vi "LVFunction_Determine if config file needs installer.vi"(0 "Config file path":path, 5 "Product version":string, 7 "Product name":string, 11 "error in (no error)":errorcluster) -> (4 "Config file path (dup)":path, 6 "must install":bool, 15 "error out":errorcluster)   [LabVIEW 2020]
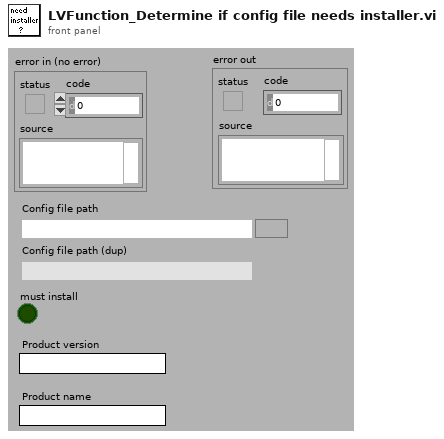
[diagram p1: front panel]
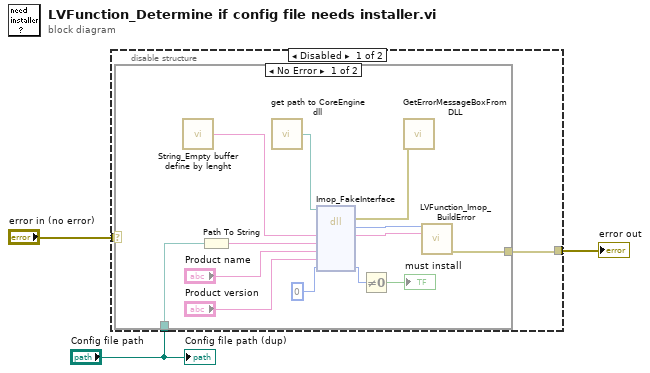
[diagram p0: block diagram]
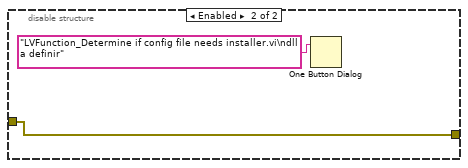
[diagram p3: hidden frame]
diagram:
  n1 = disable-structure shown="Disabled" {
    disable-tunnel: "error in (no error)" -> [w6 w22]
    disable-tunnel: "Config file path" -> [w5 _]
    disable-tunnel: [w4 w22] -> w1
    frame Disabled {
      n2 = case shown="No Error" w6 {
        selector: w6 -> [_ w20]
        tunnel: [w17 w20] -> w4
        tunnel: w5 -> [w15 _]
        frame No Error {
          n3 = call "String_Empty buffer define by lenght.vi"() -> ("Empty buffer"=w9:string)  [unwired: 1 in]
          n4 = Path To String(path=w15) -> (string=w16:string)
          n5 = call "get path to CoreEngine dll.vi"() -> ("path to wavekit library"=w7:path)  [unwired: 14 in, 1 out]
          n6 = dll-call lib="D:/SOFTware/HASO_v3/SVN_trunk/ImOpCoreEngine4_LV2011/DLLs/c_interface_vc100.dll" fn="Imop_FakeInterface"(path in=w7, "message"=w9, "config file path"=w16, "product_name"="Product name", "product_version"="Product version", "must install"=u16 0) -> (error out=w8:errorcluster, "return type"=w19:i32, "message"=w18:string, "must install"=w10:u16)  [unwired: 5 in, 1 out]
          n7 = Not Equal To 0?(x=w10) -> (x != 0?=→"must install":bool)
          n8 = call "GetErrorMessageBoxFromDLL.vi"("error IN"=w8) -> ()  [unwired: 10 in, 1 out]
          n9 = call "LVFunction_Imop_BuildError.vi"("code"=w19, "String to Prepend to source (\"\")"=w18) -> ("error out"=w17:errorcluster)  [unwired: 13 in]
        }
        frame Error {
        }
      }
    }
    frame Enabled {
      n10 = One Button Dialog(message="LVFunction_Determine if config file needs installer.vi\ndll a definir") -> ()  [unwired: 1 in, 1 out]
    }
  }
  "error out" <- w1
  "Config file path (dup)" <- "Config file path"
